vi "7-3 smoothing.vi"() -> ()   [LabVIEW 2012]
panel:
  in  "Boolean 2":bool
  out "Waveform Graph\nreal time":dbl[](graph)
  in  "Boolean":bool
  out "Waveform Graph\nvettore":cluster{i32, i32, dbl[][]}(graph)
  # "IMPLEMENTARE LO  SMOOTING (vettore e real-time)  SU TRE \nVALORI IN USCITA AD UN GENERATORE DI NUMERI CASUALI. \n VISUALIZZARE IL RISULTATO CON IL DATO ORIGINALE IN\nUN GRAFICO ABILITANDO CURSORI etc."
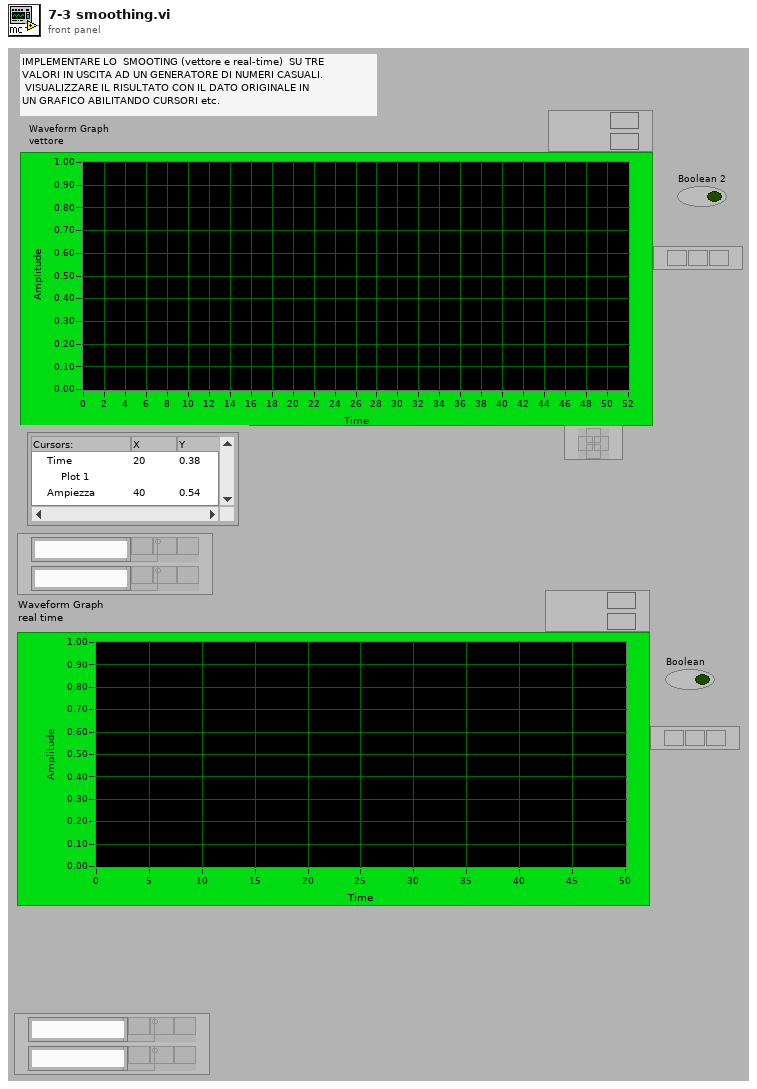
[diagram p1: front panel]
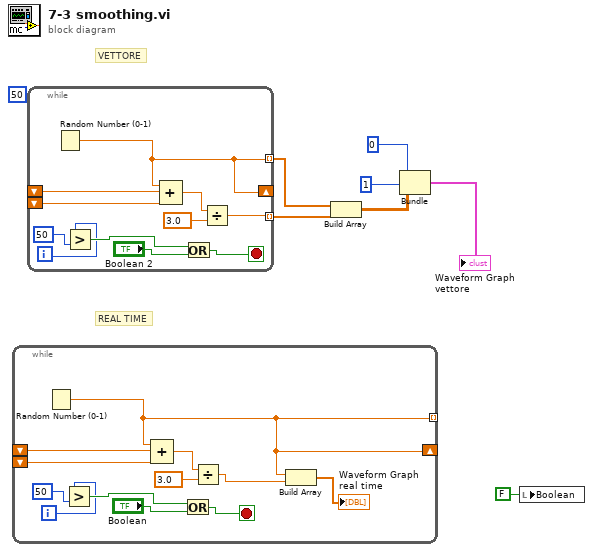
[diagram p0: block diagram]
diagram:
  (unwired) 50
  # "REAL TIME"
  # "VETTORE"
  n1 = while {
    shift-right: [w8] -> _
    shift-left: _ -> [w18]
    shift-left: _ -> [w17]
    tunnel: [w8] -> _ mode=indexing
    i -> [w11]
    stop <- w13 stop-if-true
    n2 = Random Number (0-1)() -> (number: 0 to 1=w8:dbl)
    n3 = Greater?(x=w11, y=50 ("x")) -> (0:w14:bool)
    n4 = Compound Arithmetic op=ADD(w8, w18, w17) -> (w16:dbl)
    n5 = Or(x=w14, y="Boolean") -> (x .or. y?=w13:bool)
    n6 = Divide(x=w16, y=3.0) -> (x/y=w9:dbl)
    n7 = Build Array(w8, w9) -> (→"Waveform Graph\nreal time":dbl[])
  }
  n8 = while {
    shift-right: [w25] -> _
    shift-left: _ -> [w28]
    shift-left: _ -> [w27]
    tunnel: [w29] -> w3 mode=indexing
    tunnel: [w25] -> w4 mode=indexing
    i -> [w21]
    stop <- w20 stop-if-true
    n9 = Random Number (0-1)() -> (number: 0 to 1=w25:dbl)
    n10 = Greater?(x=w21, y=50 ("x")) -> (0:w23:bool)
    n11 = Compound Arithmetic op=ADD(w25, w28, w27) -> (w26:dbl)
    n12 = Or(x=w23, y="Boolean 2") -> (x .or. y?=w20:bool)
    n13 = Divide(x=w26, y=3.0) -> (x/y=w29:dbl)
  }
  n14 = Build Array(w4, w3) -> (w5:dbl[][])
  n15 = Bundle(0, 1, w5) -> (→"Waveform Graph\nvettore":cluster{i32, i32, dbl[][]})  [unwired: 1 in]
  n16 = local write "Boolean"(FALSE ("Boolean")) -> ()
